vi "Do.vi"(8 "error in (no error)":errorcluster, 10 "Actor in":refnum<class "Actor.lvclass">, 11 "Load Measurements Message":refnum<class "Find Measurements On Disk Message.lvclass">) -> (0 "error out":errorcluster, 2 "Actor out":refnum<class "Actor.lvclass">)   [LabVIEW 2015, in "Controller Actor.lvlib" / "Find Measurements On Disk Message.lvclass"]
uses:
  Find Measurements On Disk Message.lvclass
  <vilib>/ActorFramework/Actor/Actor.lvclass
  Controller.lvclass
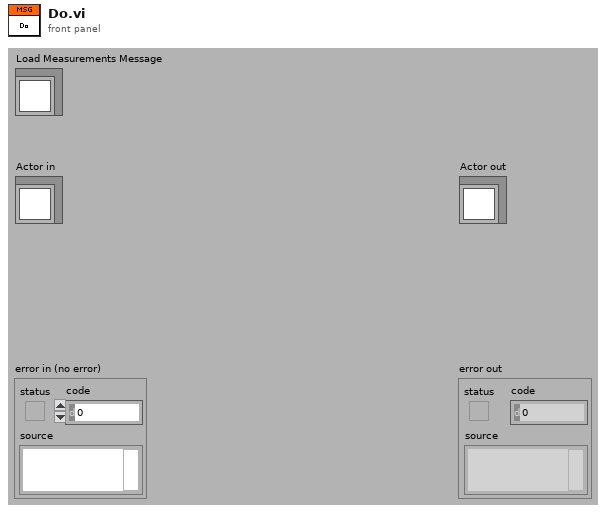
[diagram p1: front panel]
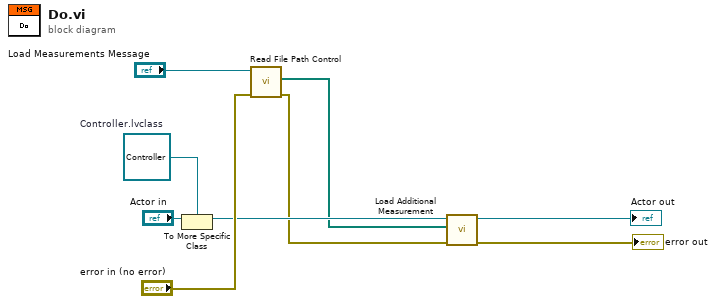
[diagram p0: block diagram]
diagram:
  w7 = refnum<class "Controller.lvclass"> refnum  # Controller.lvclass
  n1 = To More Specific Class(target class=w7, reference="Actor in") -> (specific class reference=w5:refnum<class "Controller.lvclass">)  [unwired: 1 in, 1 out]
  n2 = call "Read File Path Control.vi"("error in (no error)"="error in (no error)", "Load Measurements Message in"="Load Measurements Message") -> ("error out"=w4:errorcluster, "Array of Measurement Paths"=w3:path[])  [unwired: 7 in, 1 out]
  n3 = call "Load Additional Measurement.vi"("error in (no error)"=w4, "Array of Measurement Paths"=w3, "Controller in"=w5) -> ("error out"=→"error out":errorcluster, "Controller out"=→"Actor out":refnum<class "Controller.lvclass">)  [unwired: 7 in]
